vi "TreeNodeArray Destroy.vi"(8 "error in (no error)":errorcluster, 11 "TreeNodeArray DVR in":refnum<data-value>) -> (0 "error out":errorcluster)   [LabVIEW 2012, in "MDSplus.lvlib"]
uses:
  <vilib>/MDSplus/Library/MDSplus.lvlib
  <vilib>/MDSplus/Classes/TreeNodeArray_Class/TreeNodeArray.lvclass
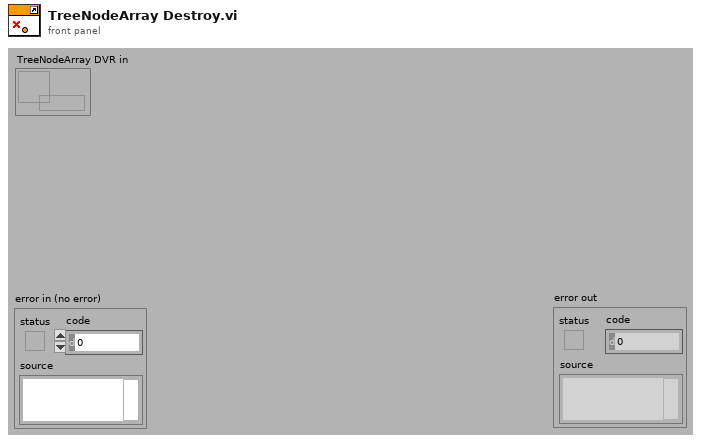
[diagram p1: front panel]
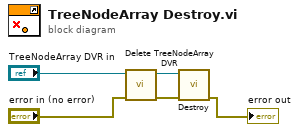
[diagram p0: block diagram]
diagram:
  n1 = call <vilib>:"Delete TreeNodeArray DVR.vi"("error in (no error)"="error in (no error)", "TreeNodeArray DVR in"="TreeNodeArray DVR in") -> ("error out"=w2:errorcluster, "TreeNodeArray out"=w3:refnum<class "TreeNodeArray.lvclass">)  [unwired: 8 in]
  n2 = call-dynamic "Destroy.vi"("error in (no error)"=w2, "TreeNodeArray in"=w3) -> ("error out"=→"error out":errorcluster)  [unwired: 9 in]
